vi "Update Build Version.vi"(8 "error in (no error)":errorcluster, 11 "PostBuildSupport in":refnum<class "PostBuildSupport.lvclass">) -> (0 "error out":errorcluster, 3 "PostBuildSupport out":refnum<class "PostBuildSupport.lvclass">)   [LabVIEW 2019, in "PostBuildSupport.lvclass"]
uses:
  PostBuildSupport.lvclass
  PostBuildSupport.lvclass/PostBuildSupport.ctl
  <vilib>/AppBuilder/AB_API_Simple/Set Build Specification Version (path).vi
  <vilib>/AppBuilder/AB_API_Simple/NI_App_Builder_API.lvlib
  Build/Build.lvlib
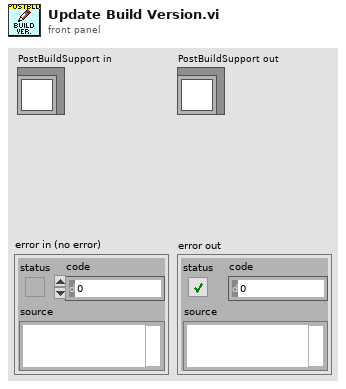
[diagram p1: front panel]
types:
  T1 = typedef "NI_App_Builder_API.lvlib/Build Specification Version.ctl" = cluster{"Major":u16, "Minor":u16, "Fix":u16, "Build":u16}
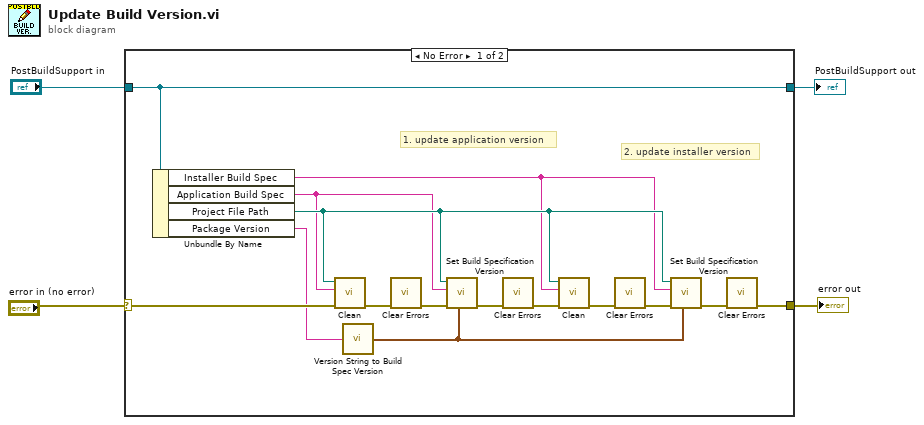
[diagram p0: block diagram]
diagram:
  n1 = case shown="No Error" "error in (no error)" {
    selector: "error in (no error)" -> [w18 w20]
    tunnel: [w10 w20] -> w4
    tunnel: "PostBuildSupport in" -> [w19 w21]
    tunnel: [w19 w21] -> w2
    frame No Error {
      # "2. update installer version"
      # "1. update application version"
      n2 = Unbundle By Name(w19) -> ("Installer Build Spec"=w5:string, "Application Build Spec"=w6:string, "Project File Path"=w7:path, "Package Version"=w9:string)
      n3 = call <vilib>:"Clean.vi"("error in (no error)"=w18, "Name of build specification (if empty: clean all)"=w6, "Path to project"=w7) -> ("error out"=w14:errorcluster)  [unwired: 8 in]
      n4 = call "Version String to Build Spec Version.vi"("Package Version"=w9) -> ("Build Specification Version"=w8:T1)
      n5 = call <vilib>:"Clear Errors.vi"("error in (no error)"=w14) -> ("error out"=w17:errorcluster)  [unwired: 5 in, 1 out]
      n6 = call-poly <vilib>:"Set Build Specification Version.vi"("Build Specification Version"=w8, "error in (no error)"=w17, "Name of build specification"=w6, "Path to project"=w7) -> ("error out"=w16:errorcluster)  [unwired: 7 in]
      n7 = call <vilib>:"Clear Errors.vi"("error in (no error)"=w16) -> ("error out"=w15:errorcluster)  [unwired: 5 in, 1 out]
      n8 = call <vilib>:"Clean.vi"("error in (no error)"=w15, "Name of build specification (if empty: clean all)"=w5, "Path to project"=w7) -> ("error out"=w13:errorcluster)  [unwired: 8 in]
      n9 = call <vilib>:"Clear Errors.vi"("error in (no error)"=w13) -> ("error out"=w12:errorcluster)  [unwired: 5 in, 1 out]
      n10 = call-poly <vilib>:"Set Build Specification Version.vi"("Build Specification Version"=w8, "error in (no error)"=w12, "Name of build specification"=w5, "Path to project"=w7) -> ("error out"=w11:errorcluster)  [unwired: 7 in]
      n11 = call <vilib>:"Clear Errors.vi"("error in (no error)"=w11) -> ("error out"=w10:errorcluster)  [unwired: 5 in, 1 out]
    }
    frame Error {
    }
  }
  "error out" <- w4
  "PostBuildSupport out" <- w2
